vi "main_reset_panel.vi"(3 "Env ready?":refnum<vi>, 4 "Envi. Tree":refnum<vi>, 5 "Env. Directory":refnum<vi>, 6 "Iteration":refnum<vi>, 7 "Runtime":refnum<vi>, 8 "Runtime (string)":refnum<vi>, 9 "Active Element":refnum<vi>, 10 "Simulation Log":refnum<vi>, 11 "Plant Structure":refnum<vi>) -> ()   [LabVIEW 2019]
uses:
  <vilib>/Utility/sysdir.llb/System Directory Type.ctl
  lib/libSimulationControl/libSimulationControl.lvlib
panel:
  # "*******************************************************************\nBiogas Plant Control\n\nAuthor: Paul Zügel\nGCSC-Frankfurt am Main 2020\n\n*******************************************************************"
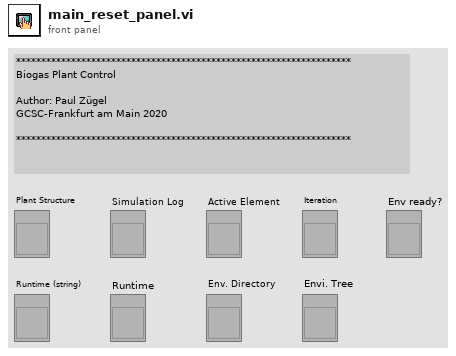
[diagram p1: front panel]
types:
  T1 = typedef "System Directory Type.ctl" = i32
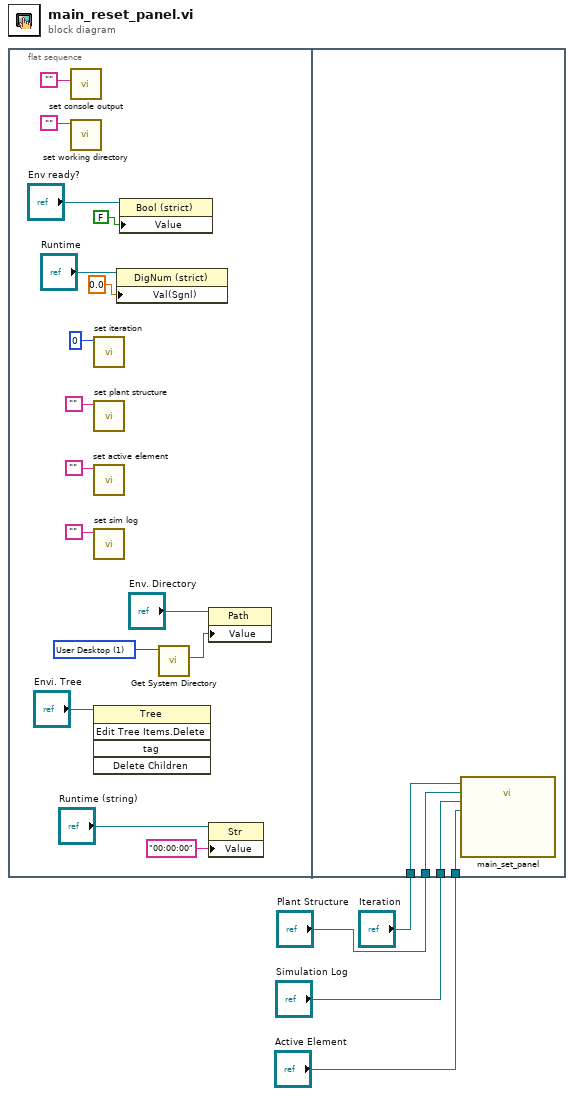
[diagram p0: block diagram]
diagram:
  n1 = flat-sequence {
    tunnel: "Plant Structure" -> [w24]
    tunnel: "Simulation Log" -> [w23]
    tunnel: "Active Element" -> [w22]
    tunnel: "Iteration" -> [w21]
    frame #0 {
      w10 = T1 1 items=["User Home"=0, "User Desktop"=1, "User Documents"=2, "User Application Data"=3, "User Preferences"=4, "User Temporary"=5, "Public Documents"=6, "Public Application Data"=7, "Public Preferences"=8, "Public Cache"=13, "System Core Libraries"=9, "System Installed Libraries"=10, "Application Files"=11, "Boot Volume Root"=12] ("system directory type")
      n2 = call "set console output.vi"("console_output"="") -> ()  [unwired: 11 in]
      n3 = call "set working directory.vi"("dir"="") -> ()  [unwired: 10 in, 1 out]
      n4 = call "set iteration.vi"("iter"=0 ("Value")) -> ()  [unwired: 10 in, 1 out]
      n5 = call "set plant structure.vi"("structure"="") -> ()  [unwired: 10 in, 1 out]
      n6 = call "set active element.vi"("elem"="") -> ()  [unwired: 10 in, 1 out]
      n7 = call "set sim log.vi"("log"="") -> ()  [unwired: 10 in, 1 out]
      n8 = invoke on="Invoke Node" class="Tree" method="Edit Tree Items.Delete"(reference="Envi. Tree") -> ()  [unwired: 4 in, 5 out]
      n9 = property on="Property Node" class="DigNum (strict)"(reference="Runtime", "Val(Sgnl)"=0.0 ("Value (Signaling)")) -> ()  [unwired: 1 in, 2 out]
      n10 = property class="Bool (strict)"(reference="Env ready?", "Value"=FALSE) -> ()  [unwired: 1 in, 2 out]
      n11 = call <vilib>:"Get System Directory.vi"("system directory type"=w10) -> ("system directory"=w11:path)  [unwired: 10 in]
      n12 = property on="Property Node" class="Path"(reference="Env. Directory", "Value"=w11) -> ()  [unwired: 1 in, 2 out]
      n13 = property on="Property Node" class="Str"(reference="Runtime (string)", "Value"="00:00:00") -> ()  [unwired: 1 in, 2 out]
    }
    frame #1 {
      n14 = call "main_set_panel.vi"("Active Element"=w22, "Simulation Log"=w23, "Plant Structure"=w24, "Iteration"=w21) -> ()  [unwired: 8 in]
    }
  }
